vi "Reader Page.vi"(8 "error in (no error)":errorcluster, 11 "Node Ptr":T2 format="%.0x") -> (0 "error out":errorcluster)   [LabVIEW 2016, in "DDS Custom Device System Explorer.lvlib"]
uses:
  DDS Custom Device System Explorer.lvlib
  <vilib>/NI Veristand/Custom Device API/Custom Device Item Ref.ctl
  Shared/key Enum.ctl
  <vilib>/NI VeriStand/Custom Device API/Custom Device API.lvlib
  Shared/DDS Custom Device Shared.lvlib
panel:
  in  "Default Key":T1
  in  "Force Read (only for Exclusive Reader)?":bool
  in  "Force Exclusive Reader?":bool
  in  "Data Writer QoS Profile":string
  in  "Domain Participant QoS Profile":string
  in  "Type Name":string
  in  "Domain id":u32
  in  "Topic Name":string
  in  "SHDocVw.IWebBrowser":refnum<k7>(container)
  in  "General Header":cluster{"Section Name":string}={"Section Name"="General Custom Device Settings"}
  in  "Description":string
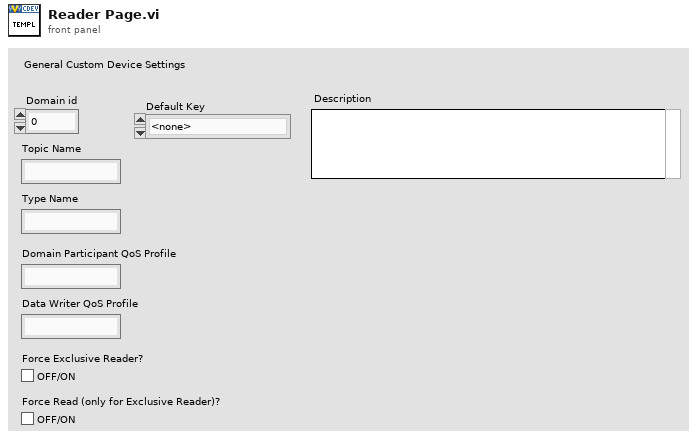
[diagram p1: front panel]
types:
  T1 = typedef "DDS Custom Device Shared.lvlib/key Enum.ctl" = enum16{"<none>", "I32_Num", "I64_Num", "U16_Num", "innercluster.Sgl_Num", "innercluster.Boolean"}
  T2 = typedef "Custom Device API.lvlib/Custom Device Item Ref.ctl" = u64
  T3 = typedef "DDS Custom Device Shared.lvlib/WriterReaderConfiguration.ctl" = cluster{"Topic Name":string, "Domain Id":u32, "Advanced Configuration":T4}
  T4 = typedef "DDS Custom Device Shared.lvlib/Advanced DDS Configuration.ctl" = cluster{"typeName":string, "key Name":T1, "domainParticipantQoSProfile":string, "dataWriterQoSProfile":string, "forceArrayMapping?":bool, "forceUnboundedString?":bool, "forceExclusiveReader?":bool, "forceRead? (only ExclusiveReader)":bool, "ContentFilteredTopic Info":T5}
  T5 = typedef "LVDDS_library.lvlib/RTI DDS ContentFilteredTopic Info.ctl" = cluster{"Filter Type":string, "ContentFilteredTopic Name":string, "Filter Expression":string}
  T6 = typedef "Custom Device API.lvlib/Custom Device Commands.ctl" = enum16{"Default", "Item renamed", "Shutdown", "Dynamic button pressed"}
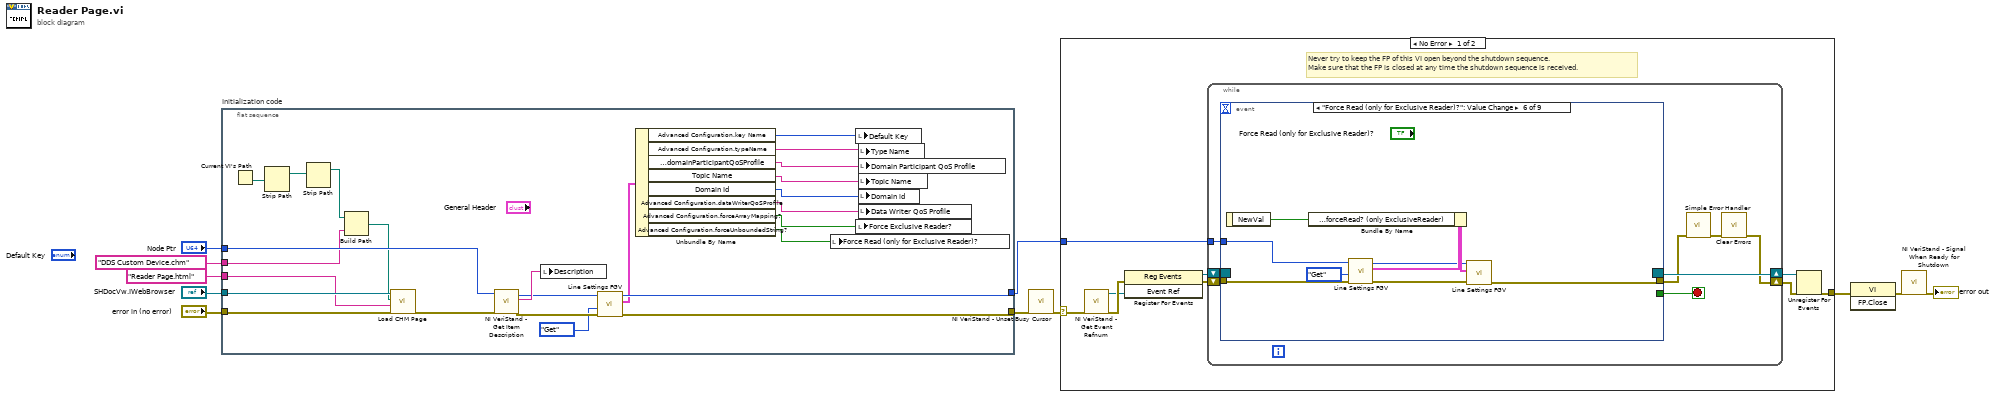
[diagram p0: block diagram]
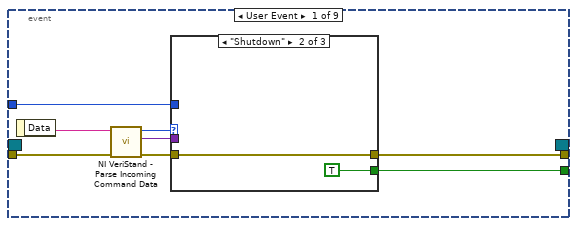
[diagram p2: hidden frame]
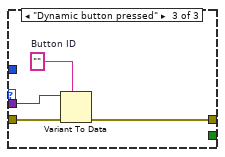
[diagram p4: hidden frame]
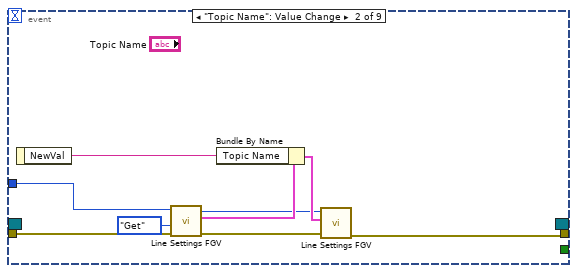
[diagram p5: hidden frame]
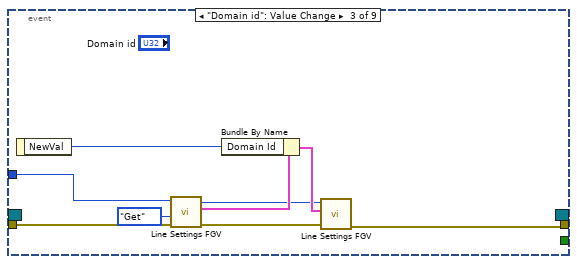
[diagram p6: hidden frame]
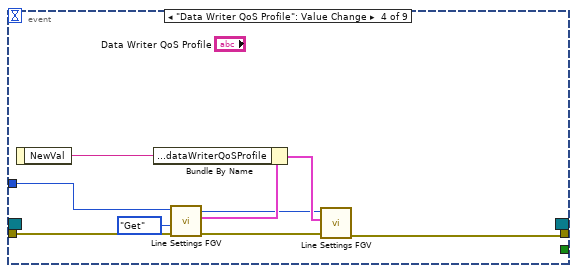
[diagram p7: hidden frame]
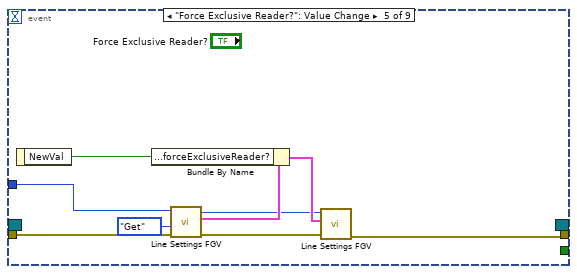
[diagram p8: hidden frame]
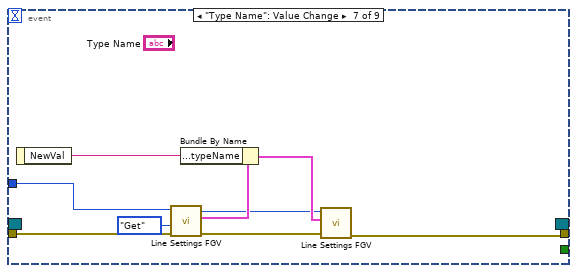
[diagram p9: hidden frame]
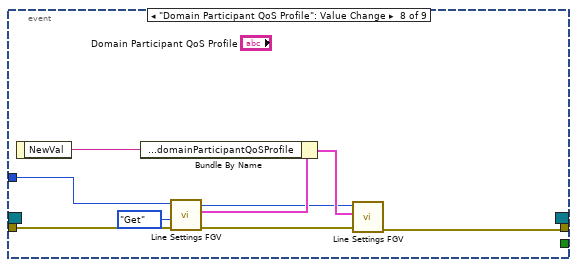
[diagram p10: hidden frame]
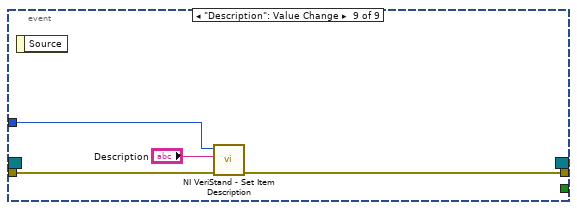
[diagram p11: hidden frame]
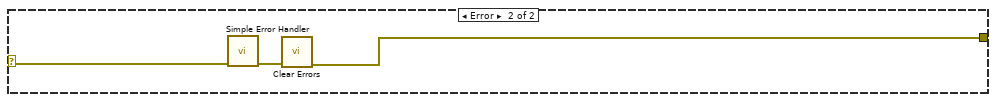
[diagram p12: hidden frame]
diagram:
  n1 = flat-sequence "Initialization code" {
    tunnel: "error in (no error)" -> [w20]
    tunnel: "Node Ptr" -> [w36]
    tunnel: [w31] -> w7
    tunnel: [w30] -> w4
    tunnel: "SHDocVw.IWebBrowser" -> [w18]
    tunnel: "Reader Page.html" ("HTML File") -> [w17]
    tunnel: "DDS Custom Device.chm" ("CD_CHM_FileName") -> [w13]
    frame #0 {
      n2 = Current VI's Path() -> (path=w14:path)
      n3 = Strip Path(path=w14) -> (stripped path=w15:path)  [unwired: 1 out]
      n4 = Strip Path(path=w15) -> (stripped path=w16:path)  [unwired: 1 out]
      n5 = Build Path(base path=w16, name or relative path=w13) -> (appended path=w12:path)
      n6 = call <vilib>:"Load CHM Page.vi"("error in (no error)"=w20, "HTML File"=w17, "Compiled CHM Path"=w12, "Web Browser Reference"=w18) -> ("error out"=w19:errorcluster)  [unwired: 7 in]
      n7 = call <vilib>:"NI VeriStand - Get Item Description.vi"("error in (no error)"=w19, "Item Ref in"=w36) -> ("error out"=w34:errorcluster, "Description"=w35:string, "Item Ref out"=w33:T2)  [unwired: 7 out]
      n8 = local write "Description"(w35) -> ()
      n9 = call "Line Settings FGV.vi"("error in (no error)"=w34, "Get/Set"=enum16{"Set", "Get"}."Get", "Item Ref in"=w33) -> ("error out"=w31:errorcluster, "Line"=w29:T3, "Item Ref out"=w30:T2)  [unwired: 6 in]
      n10 = Unbundle By Name(w29) -> ("Advanced Configuration.key Name"=w28:T1, "Advanced Configuration.typeName"=w27:string, "Advanced Configuration.domainParticipantQoSProfile"=w26:string, "Topic Name"=w25:string, "Domain Id"=w24:u32, "Advanced Configuration.dataWriterQoSProfile"=w23:string, "Advanced Configuration.forceArrayMapping?"=w22:bool, "Advanced Configuration.forceUnboundedString?"=w21:bool)
      n11 = local write "Force Read (only for Exclusive Reader)?"(w21) -> ()
      n12 = local write "Default Key"(w28) -> ()
      n13 = local write "Force Exclusive Reader?"(w22) -> ()
      n14 = local write "Type Name"(w27) -> ()
      n15 = local write "Domain Participant QoS Profile"(w26) -> ()
      n16 = local write "Topic Name"(w25) -> ()
      n17 = local write "Domain id"(w24) -> ()
      n18 = local write "Data Writer QoS Profile"(w23) -> ()
    }
  }
  n19 = call <vilib>:"NI VeriStand - Unset Busy Cursor.vi"("error in (no error)"=w7) -> ("error out"=w6:errorcluster)  [unwired: 10 out]
  n20 = case shown="No Error" w6 {
    selector: w6 -> [w37 w138]
    tunnel: [w42 w136] -> w11
    tunnel: w4 -> [w38 _]
    frame No Error {
      # "Never try to keep the FP of this VI open beyond the shutdown sequence.\nMake sure that the FP is closed at any time the shutdown sequence is received."
      n21 = call <vilib>:"NI VeriStand - Get Event Refnum.vi"("error in (no error)"=w37) -> ("error out"=w45:errorcluster, "Event Ref"=w41:refnum<user-event>)  [unwired: 9 out]
      n22 = register-events(error in=w45, w41) -> (reference out=w39:refnum<event-registration>, error out=w40:errorcluster)  [unwired: 1 in]
      n23 = while {
        tunnel: w38 -> [w49]
        shift-right: [w46] -> w43
        shift-left: w40 -> [w52]
        shift-right: [w53] -> w44
        shift-left: w39 -> [w51]
        stop <- w50 stop-if-true
        n24 = event shown="[5] \"Force Read (only for Exclusive Reader)?\": Value Change" {
          selector: w51 -> [_ _ _ _ _ _ _ _ _]
          dyn-events: [_ _ _ _ _ _ _ _ _] -> w53
          timeout: _ -> [_ _ _ _ _ _ _ _ _]
          tunnel: w52 -> [w61 w77 w86 w95 w104 w113 w122 w131 w134]
          tunnel: [w57 _ _ _ _ _ _ _ _] -> w50
          tunnel: [w56 w69 w78 w87 w96 w105 w114 w123 w133] -> w48
          tunnel: w49 -> [w55 w76 w85 w94 w103 w112 w121 w130 w135]
          event User Event {
            n25 = event-data() -> ("Data"=w60:string)  [unwired: 1 out]
            n26 = call <vilib>:"NI VeriStand - Parse Incoming Command Data.vi"("error in (no error)"=w61, "Incoming data"=w60) -> ("error out"=w59:errorcluster, "Outgoing data"=w54:variant, "Action"=w58:T6)  [unwired: 7 out]
            n27 = case shown="\"Shutdown\"" w58 {
              tunnel: w59 -> [w62 w63 w68]
              tunnel: [_ TRUE _] -> w57
              tunnel: [w62 w63 w65] -> w56
              tunnel: w55 -> [_ _ _]
              tunnel: w54 -> [_ _ w67]
              frame "Default", Default {
              }
              frame "Shutdown" {
              }
              frame "Dynamic button pressed" {
                w66 = ""  # Button ID
                n28 = Variant To Data(error in=w68, type=w66, Variant=w67) -> (error out=w65:errorcluster)  [unwired: 1 out]
              }
            }
          }
          event "Topic Name": Value Change {
            n29 = event-data() -> ("NewVal"=w72:string)  [unwired: 1 out]
            n30 = call "Line Settings FGV.vi"("error in (no error)"=w77, "Get/Set"=enum16{"Set", "Get"}."Get", "Item Ref in"=w76) -> ("error out"=w74:errorcluster, "Line"=w73:T3, "Item Ref out"=w70:T2)  [unwired: 6 in]
            n31 = Bundle By Name(cluster=w73, "Topic Name"=w72) -> (w71:T3)
            n32 = call "Line Settings FGV.vi"("error in (no error)"=w74, "Line"=w71, "Item Ref in"=w70) -> ("error out"=w69:errorcluster)  [unwired: 6 in, 2 out]
          }
          event "Domain id": Value Change {
            n33 = event-data() -> ("NewVal"=w81:u32)  [unwired: 1 out]
            n34 = call "Line Settings FGV.vi"("error in (no error)"=w86, "Get/Set"=enum16{"Set", "Get"}."Get", "Item Ref in"=w85) -> ("error out"=w83:errorcluster, "Line"=w82:T3, "Item Ref out"=w79:T2)  [unwired: 6 in]
            n35 = Bundle By Name(cluster=w82, "Domain Id"=w81) -> (w80:T3)
            n36 = call "Line Settings FGV.vi"("error in (no error)"=w83, "Line"=w80, "Item Ref in"=w79) -> ("error out"=w78:errorcluster)  [unwired: 6 in, 2 out]
          }
          event "Data Writer QoS Profile": Value Change {
            n37 = event-data() -> ("NewVal"=w90:string)  [unwired: 1 out]
            n38 = call "Line Settings FGV.vi"("error in (no error)"=w95, "Get/Set"=enum16{"Set", "Get"}."Get", "Item Ref in"=w94) -> ("error out"=w92:errorcluster, "Line"=w91:T3, "Item Ref out"=w88:T2)  [unwired: 6 in]
            n39 = Bundle By Name(cluster=w91, "Advanced Configuration.dataWriterQoSProfile"=w90) -> (w89:T3)
            n40 = call "Line Settings FGV.vi"("error in (no error)"=w92, "Line"=w89, "Item Ref in"=w88) -> ("error out"=w87:errorcluster)  [unwired: 6 in, 2 out]
          }
          event "Force Exclusive Reader?": Value Change {
            n41 = event-data() -> ("NewVal"=w99:bool)  [unwired: 1 out]
            n42 = call "Line Settings FGV.vi"("error in (no error)"=w104, "Get/Set"=enum16{"Set", "Get"}."Get", "Item Ref in"=w103) -> ("error out"=w101:errorcluster, "Line"=w100:T3, "Item Ref out"=w97:T2)  [unwired: 6 in]
            n43 = Bundle By Name(cluster=w100, "Advanced Configuration.forceExclusiveReader?"=w99) -> (w98:T3)
            n44 = call "Line Settings FGV.vi"("error in (no error)"=w101, "Line"=w98, "Item Ref in"=w97) -> ("error out"=w96:errorcluster)  [unwired: 6 in, 2 out]
          }
          event "Force Read (only for Exclusive Reader)?": Value Change {
            n45 = event-data() -> ("NewVal"=w108:bool)  [unwired: 1 out]
            n46 = call "Line Settings FGV.vi"("error in (no error)"=w113, "Get/Set"=enum16{"Set", "Get"}."Get", "Item Ref in"=w112) -> ("error out"=w110:errorcluster, "Line"=w109:T3, "Item Ref out"=w106:T2)  [unwired: 6 in]
            n47 = Bundle By Name(cluster=w109, "Advanced Configuration.forceRead? (only ExclusiveReader)"=w108) -> (w107:T3)
            n48 = call "Line Settings FGV.vi"("error in (no error)"=w110, "Line"=w107, "Item Ref in"=w106) -> ("error out"=w105:errorcluster)  [unwired: 6 in, 2 out]
          }
          event "Type Name": Value Change {
            n49 = event-data() -> ("NewVal"=w117:string)  [unwired: 1 out]
            n50 = call "Line Settings FGV.vi"("error in (no error)"=w122, "Get/Set"=enum16{"Set", "Get"}."Get", "Item Ref in"=w121) -> ("error out"=w119:errorcluster, "Line"=w118:T3, "Item Ref out"=w115:T2)  [unwired: 6 in]
            n51 = Bundle By Name(cluster=w118, "Advanced Configuration.typeName"=w117) -> (w116:T3)
            n52 = call "Line Settings FGV.vi"("error in (no error)"=w119, "Line"=w116, "Item Ref in"=w115) -> ("error out"=w114:errorcluster)  [unwired: 6 in, 2 out]
          }
          event "Domain Participant QoS Profile": Value Change {
            n53 = event-data() -> ("NewVal"=w126:string)  [unwired: 1 out]
            n54 = call "Line Settings FGV.vi"("error in (no error)"=w131, "Get/Set"=enum16{"Set", "Get"}."Get", "Item Ref in"=w130) -> ("error out"=w128:errorcluster, "Line"=w127:T3, "Item Ref out"=w124:T2)  [unwired: 6 in]
            n55 = Bundle By Name(cluster=w127, "Advanced Configuration.domainParticipantQoSProfile"=w126) -> (w125:T3)
            n56 = call "Line Settings FGV.vi"("error in (no error)"=w128, "Line"=w125, "Item Ref in"=w124) -> ("error out"=w123:errorcluster)  [unwired: 6 in, 2 out]
          }
          event "Description": Value Change {
            n57 = event-data() -> ()  [unwired: 2 out]
            n58 = call <vilib>:"NI VeriStand - Set Item Description.vi"("error in (no error)"=w134, "Description"="Description", "Item Ref in"=w135) -> ("error out"=w133:errorcluster)  [unwired: 8 out]
          }
        }
        n59 = call <vilib>:"Simple Error Handler.vi"("error in (no error)"=w48) -> ("error out"=w47:errorcluster)  [unwired: 1 in, 7 out]
        n60 = call <vilib>:"Clear Errors.vi"("error in (no error)"=w47) -> ("error out"=w46:errorcluster)  [unwired: 1 in, 5 out]
      }
      n61 = Unregister For Events(event registration refnum=w44, error in=w43) -> (error out=w42:errorcluster)
    }
    frame Error {
      n62 = call <vilib>:"Simple Error Handler.vi"("error in (no error)"=w138) -> ("error out"=w137:errorcluster)  [unwired: 1 in, 7 out]
      n63 = call <vilib>:"Clear Errors.vi"("error in (no error)"=w137) -> ("error out"=w136:errorcluster)  [unwired: 1 in, 5 out]
    }
  }
  n64 = invoke class="VI" method="FP.Close"(error in=w11) -> (error out=w10:errorcluster)  [unwired: 2 in, 2 out]
  n65 = call <vilib>:"NI VeriStand - Signal When Ready for Shutdown.vi"("error in (no error)"=w10) -> ("error out"=→"error out":errorcluster)  [unwired: 10 out]
